vi "PythonBDConverter.vi"(5 "Build Directory":path, 6 "error in":errorcluster, 9 "VI Interpreter in":refnum<class "VI Interpreter.lvclass">) -> (0 "error out":errorcluster, 3 "PythonConverter out":refnum<class "PythonBDConverter.lvclass">)   [LabVIEW 2014, in "PythonBDConverter.lvclass"]
uses:
  PythonBDConverter.lvclass
  VI Interpreter/Classes/VI Interpreter/VI Interpreter.lvclass
  PythonBDConverter.lvclass/PythonBDConverter.ctl
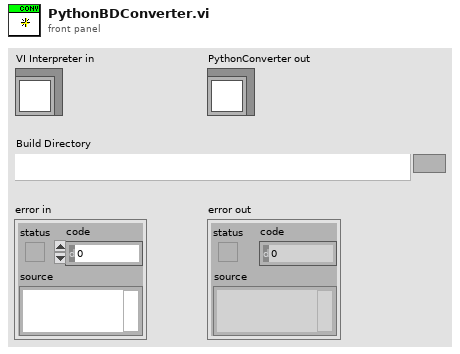
[diagram p1: front panel]
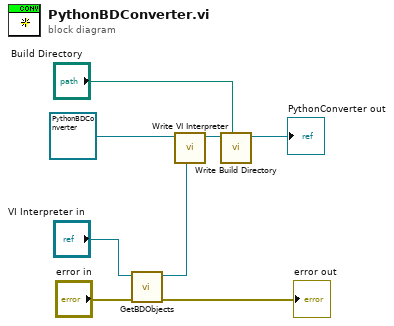
[diagram p0: block diagram]
diagram:
  n1 = call "GetBDObjects.vi"("error in"="error in", "VI Interpreter in"="VI Interpreter in") -> ("error out"=→"error out":errorcluster, "VI Interpreter out"=w5:refnum<class "VI Interpreter.lvclass">)  [unwired: 8 in]
  n2 = call "Write VI Interpreter.vi"("VI Interpreter"=w5, "PythonConverter_BD in"=refnum<class "PythonBDConverter.lvclass"> refnum ("PythonConverter in")) -> ("PythonConverter_BD out"=w4:refnum<class "PythonBDConverter.lvclass">)  [unwired: 7 in]
  n3 = call "Write Build Directory.vi"("Build Directory"="Build Directory", "PythonConverter_BD in"=w4) -> ("PythonConverter_BD out"=→"PythonConverter out":refnum<class "PythonBDConverter.lvclass">)  [unwired: 7 in]
